vi "ReadFlagImpairConfig.vi"(8 "error in (no error)":errorcluster, 9 "clFlagImpairConfig":T1, 10 "ModuleID":i32) -> (0 "error out":errorcluster)   [LabVIEW 2014, in "FlagImpairModule.lvlib"]
uses:
  FlagImpairModule.lvlib
  PublicAPI/Arguments/Requests/clFlagImpairConfig.ctl
  clEventType.ctl
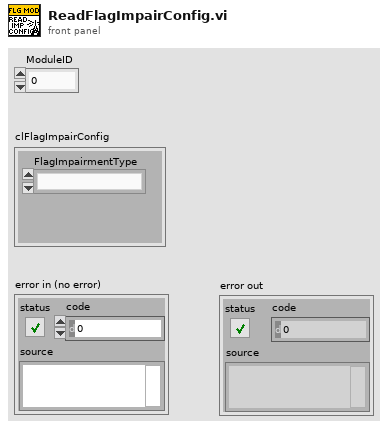
[diagram p1: front panel]
types:
  T1 = typedef "FlagImpairModule.lvlib/clFlagImpairConfig.ctl" = cluster{"FlagImpairmentType":u16}
  T2 = typedef "FlagImpairModule.lvlib/clEventType.ctl" = cluster{"ModuleID":i32, "Data":variant}
  T3 = typedef "FlagImpairModule.lvlib/clBroadcastEvents.ctl" = cluster{"DidInit":refnum<user-event>, "StatusUpdate":refnum<user-event>, "ErrorReport":refnum<user-event>, "DidStop":refnum<user-event>, "ReadFlagImpairConfig":refnum<user-event>, "ReadPluginINIFilePath":refnum<user-event>, "ReadFlagImpairParams":refnum<user-event>, "ReadTimeArray":refnum<user-event>, "GetFlagImpairment":refnum<user-event>}
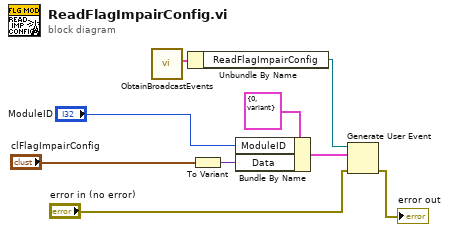
[diagram p0: block diagram]
diagram:
  n1 = call "ObtainBroadcastEvents.vi"() -> ("clBroadcastEvents"=w9:T3)  [unwired: 10 in, 1 out]
  n2 = Unbundle By Name(w9) -> ("ReadFlagImpairConfig"=w8:refnum<user-event>)
  n3 = To Variant(anything="clFlagImpairConfig") -> (Variant=w6:variant)
  n4 = Bundle By Name(cluster=T2 {"ModuleID"=0, "Data"=variant} ("clBroadcast"), "ModuleID"="ModuleID", "Data"=w6) -> (w5:T2)
  n5 = Generate User Event(user event=w8, event data cluster=w5, error in="error in (no error)") -> (error out=→"error out":errorcluster)  [unwired: 1 in, 1 out]
